vi "Customize VI Window.vi"() -> ()   [LabVIEW 2010]
doc: "이 VI는 메뉴 모음 보이기?, 제목 표시줄 보이기?, 이 VI를 가운데로와 같은 서버 메소드와 프로퍼티를 보여줍니다."
panel:
  in  "가운데":bool
  in  "정지":bool
  in  "VI를 투명하게 만들기?":bool
  in  "제목 표시줄 보이기?":bool
  in  "메뉴 모음 보이기?":bool
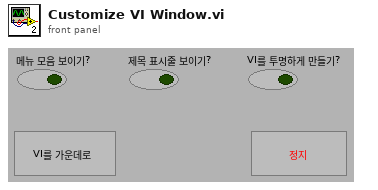
[diagram p1: front panel]
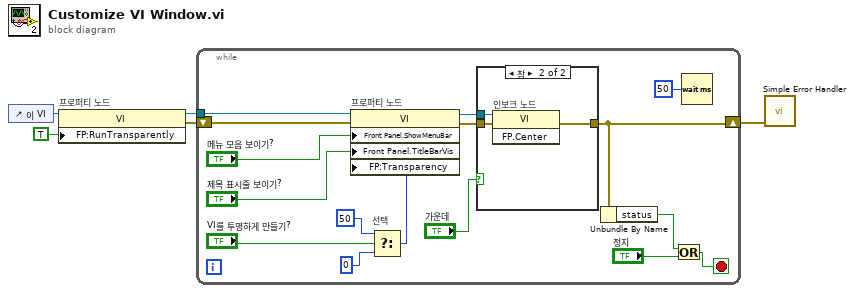
[diagram p0: block diagram]
diagram:
  n1 = control-ref of="이 VI"() -> (w5:refnum<vi>)
  n2 = property on="프로퍼티 노드" class="VI"(reference=w5, "FP:RunTransparently"=TRUE ("Front Panel Window:Run VI Transparently")) -> (reference out=w3:refnum<vi>, error out=w2:errorcluster)  [unwired: 1 in]
  n3 = while {
    tunnel: w3 -> [w21]
    shift-right: [w9] -> w1
    shift-left: w2 -> [w20]
    stop <- w10 stop-if-true
    n4 = Select "선택"(t=50, s="VI를 투명하게 만들기?", f=0) -> (s? t:f=w14:i32)
    n5 = property on="프로퍼티 노드" class="VI"(reference=w21, error in=w20, "Front Panel.ShowMenuBar"="메뉴 모음 보이기?", "Front Panel.TitleBarVis"="제목 표시줄 보이기?", "FP:Transparency"=w14) -> (reference out=w11:refnum<vi>, error out=w12:errorcluster)
    n6 = case shown="참" "가운데" {
      tunnel: w12 -> [w22 w25]
      tunnel: [w22 w24] -> w9
      tunnel: w11 -> [_ w23]
      frame False {
      }
      frame True {
        n7 = invoke on="인보크 노드" class="VI" method="FP.Center"(reference=w23, error in=w25) -> (error out=w24:errorcluster)  [unwired: 1 in, 2 out]
      }
    }
    n8 = Unbundle By Name(w9) -> ("status"=w8:bool)
    n9 = Or(x=w8, y="정지") -> (x .or. y?=w10:bool)
    n10 = Wait (ms)(milliseconds to wait=u32 50) -> ()  [unwired: 1 out]
  }
  n11 = call <vilib>:"Simple Error Handler.vi"("error in (no error)"=w1) -> ()  [unwired: 4 in, 5 out]
